vi "LoadProgram.vi"(0 "Universal Robot.lvclass in":refnum<class "Universal Robot.lvclass">, 1 "program":string, 5 "error in (no error)":errorcluster) -> (14 "Universal Robot.lvclass out":refnum<class "Universal Robot.lvclass">, 19 "error out":errorcluster)   [LabVIEW 2016, in "Universal Robot.lvclass"]
uses:
  Universal Robot.lvclass
  Universal Robot.lvclass/Universal Robot.ctl
  Client Interfaces/Dashboard Server/Dashboard Server.lvclass
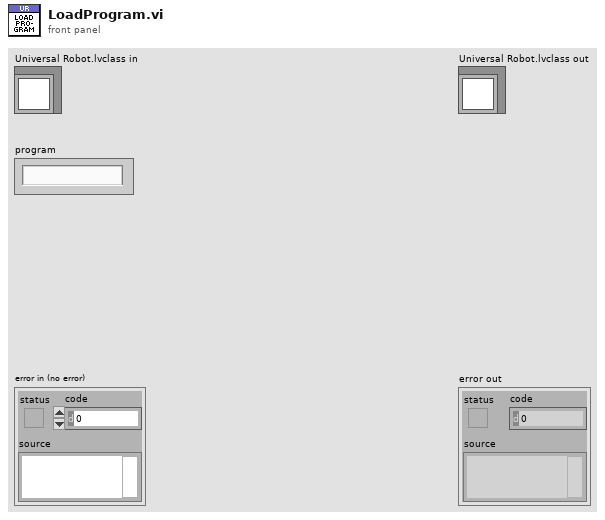
[diagram p1: front panel]
types:
  T1 = typedef "Universal Robot.lvclass/ProgramStatus.ctl" = cluster{"Loaded Program":string, "Valid Program":bool, "Program State":T2, "Running":bool}
  T2 = typedef "Universal Robot.lvclass/ProgramState.ctl" = enum16{"STOPPED", "PLAYING", "PAUSE"}
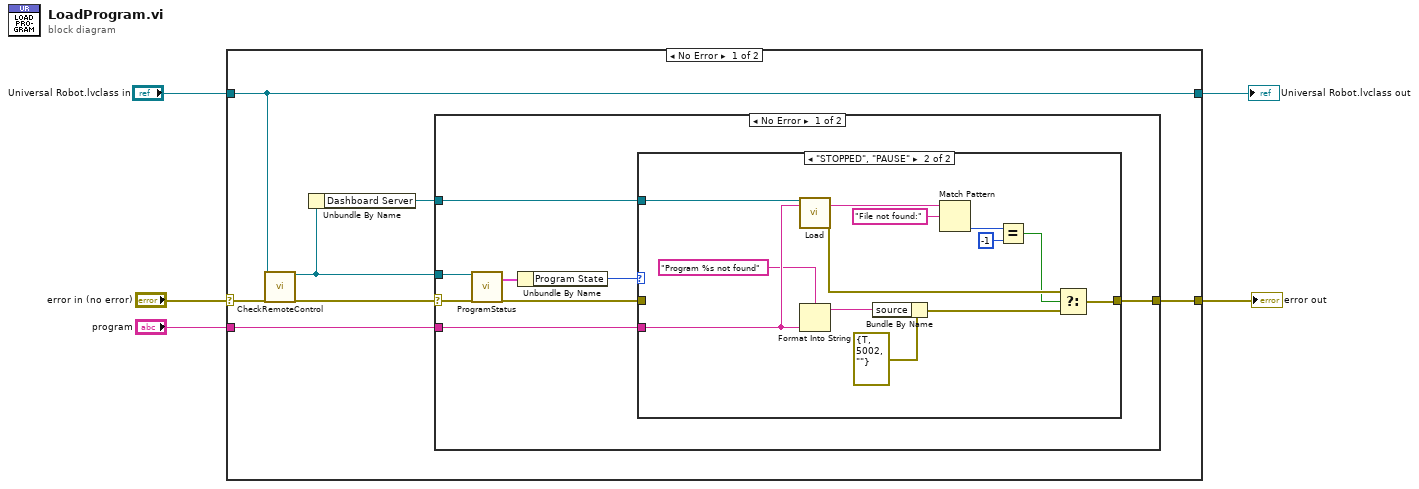
[diagram p0: block diagram]
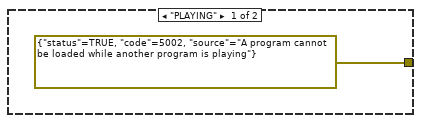
[diagram p2: hidden frame]
diagram:
  n1 = case shown="No Error" "error in (no error)" {
    selector: "error in (no error)" -> [w11 w37]
    tunnel: [w12 w37] -> w3
    tunnel: "Universal Robot.lvclass in" -> [w10 w36]
    tunnel: [w10 w36] -> w2
    tunnel: "program" -> [w7 _]
    frame No Error {
      n2 = call-dynamic "CheckRemoteControl.vi"("Universal Robot.lvclass in"=w10, "error in (no error)"=w11) -> ("Universal Robot.lvclass out"=w6:refnum<class "Universal Robot.lvclass">, "error out"=w8:errorcluster)  [unwired: 16 in]
      n3 = Unbundle By Name(w6) -> ("Dashboard Server"=w9:refnum<class "Dashboard Server.lvclass">)
      n4 = case shown="No Error" w8 {
        selector: w8 -> [w17 w35]
        tunnel: [w20 w35] -> w12
        tunnel: w9 -> [w13 _]
        tunnel: w7 -> [w19 _]
        tunnel: w6 -> [w18 _]
        frame No Error {
          n5 = call-dynamic "ProgramStatus.vi"("Universal Robot.lvclass in"=w18, "error in (no error)"=w17) -> ("Program Status"=w15:T1, "error out"=w16:errorcluster)  [unwired: 15 in, 1 out]
          n6 = Unbundle By Name(w15) -> ("Program State"=w14:T2)
          n7 = case shown="\"STOPPED\", \"PAUSE\"" w14 {
            tunnel: [errorcluster {"status"=TRUE, "code"=5002, "source"="A program cannot be loaded while another program is playing"} ("error constant") w34] -> w20
            tunnel: w19 -> [_ w25]
            tunnel: w16 -> [_ _]
            tunnel: w13 -> [_ w33]
            frame "PLAYING" {
            }
            frame "STOPPED", "PAUSE" {
              n8 = call-dynamic "Load.vi"("DashboardServer in"=w33, "program"=w25) -> ("returnStatus"=w32:string, "error out"=w28:errorcluster)  [unwired: 15 in, 1 out]
              n9 = Format Into String(format string="Program %s not found", w25) -> (resulting string=w24:string)  [unwired: 2 in, 1 out]
              n10 = Bundle By Name(cluster=errorcluster {"status"=TRUE, "code"=5002, "source"=""} ("error constant"), "source"=w24) -> (w23:errorcluster)
              n11 = Match Pattern(string=w32, regular expression="File not found:") -> (offset past match=w30:i32)  [unwired: 1 in, 3 out]
              n12 = Equal?(x=w30, y=-1) -> (x = y?=w27:bool)
              n13 = Select(t=w28, s=w27, f=w23) -> (s? t:f=w34:errorcluster)
            }
          }
        }
        frame Error {
        }
      }
    }
    frame Error {
    }
  }
  "error out" <- w3
  "Universal Robot.lvclass out" <- w2
